vi "subVI_CycleUp.vi"(8 "err in":errorcluster caption="에러 입력(에러 없음)") -> (0 "err out":errorcluster caption="에러 출력")   [LabVIEW 2016]
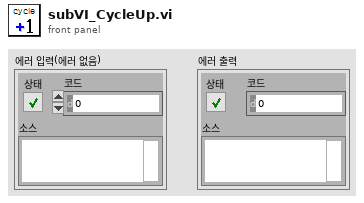
[diagram p1: front panel]
types:
  T1 = cluster{"Test Information":cluster{"date":string, "custom":string, "oper":string, "package":string, "pkg side":string, "solder":string, "brd side":string, "paste":string, "reflow":string}, "Sensor Set":cluster{"Accelerometer":cluster{"Sensitivity(mV/g)":dbl}, "Strain Guage":cluster{"Ch.":dbl[], "Gage factor":dbl[], "Resistance":dbl[], "Poisson ratio":dbl[]}}, "Resistor Set":cluster{"Criterion Level":dbl, "Res. Set":cluster{"Res. Ch":dbl, "Res. Active":bool, "Res Initial":dbl}[]}, "Test Stop Condition":cluster{"Test cycle":u16, "Fail number in a cycle":u16, "Fail factor":cluster{"Duration":u16, "Fail No.":u16}}, "Acceleration Condition ":cluster{"Shock duration pecent [%]":u16, "Filter cutoff freq":u32}, "Save":cluster{"Save Path":path, "File Name":string}}
  T2 = typedef "Total data.ctl" = cluster{"Raw Data":T3, "Resister result data":T4, "Result Table update":cluster{"Num":u32[], "Resister 1~5":u8[][], "Resister 6~10":u8[][], "Resister 11~15":u8[][]}, "Strain Data":cluster{"Strain 1":dbl, "Strain 2":dbl, "Strain 3":dbl, "Strain 4":dbl}, "Acc Result":cluster{"Acc Peak":dbl, "Acc time":dbl, "Acc area":dbl}, "STATUS":cluster{"status":string, "all_fail":bool, "emg":bool, "cycle":u16, "file name":string}, "Speed":dbl, "Acc peak time":dbl, "Max Strain":dbl, "Resistor at peak":cluster{"[0]":dbl, "[1]":dbl, "[2]":dbl, "[3]":dbl, "[4]":dbl, "[5]":dbl, "[6]":dbl, "[7]":dbl, "[8]":dbl, "[9]":dbl, "[10]":dbl, "[11]":dbl, "[12]":dbl, "[13]":dbl, "[14]":dbl}, "Acc peak index":u32, "time":string, "Cycle finish":bool, "Resistor at ini":cluster{"[0]":dbl, "[1]":dbl, "[2]":dbl, "[3]":dbl, "[4]":dbl, "[5]":dbl, "[6]":dbl, "[7]":dbl, "[8]":dbl, "[9]":dbl, "[10]":dbl, "[11]":dbl, "[12]":dbl, "[13]":dbl, "[14]":dbl}}
  T3 = typedef "raw Q data.ctl" = cluster{"Res_data":waveform(dbl)[], "Acc_data":waveform(dbl), "Strain_data":waveform(dbl)[]}
  T4 = typedef "raw data type.ctl" = cluster{"Resistor values":cluster{"[0]":dbl, "[1]":dbl, "[2]":dbl, "[3]":dbl, "[4]":dbl, "[5]":dbl, "[6]":dbl, "[7]":dbl, "[8]":dbl, "[9]":dbl, "[10]":dbl, "[11]":dbl, "[12]":dbl, "[13]":dbl, "[14]":dbl}, "Resistor tables":u8[], "Pass Fails":bool[]}
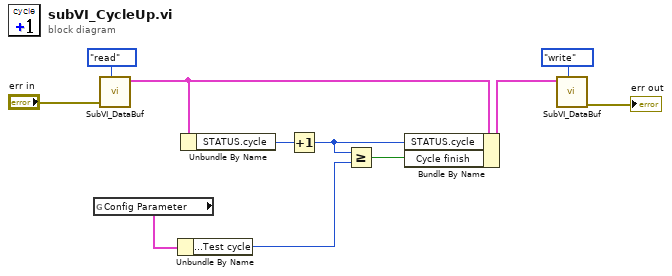
[diagram p0: block diagram]
diagram:
  n1 = global read "글로벌_Config Parameter.vi" "Config Parameter"() -> (w4:T1)
  n2 = call "SubVI_DataBuf.vi"("cmd"=enum16{"ini", "write", "read"}."read", "error in (no error)"="err in") -> ("Total data 2"=w6:T2)  [unwired: 8 in, 1 out]
  n3 = Unbundle By Name(w4) -> ("Test Stop Condition.Test cycle"=w2:u16)
  n4 = Unbundle By Name(w6) -> ("STATUS.cycle"=w9:u16)
  n5 = Increment(x=w9) -> (x+1=w3:u16)
  n6 = Greater Or Equal?(x=w3, y=w2) -> (x >= y?=w1:bool)
  n7 = Bundle By Name(cluster=w6, "STATUS.cycle"=w3, "Cycle finish"=w1) -> (w7:T2)
  n8 = call "SubVI_DataBuf.vi"("cmd"=enum16{"ini", "write", "read"}."write", "Total data"=w7) -> ("error out"=→"err out":errorcluster)  [unwired: 8 in, 1 out]
